vi "getImage.vi"(8 "error in (no error)":errorcluster, 10 "stop":bool, 11 "AndorIKonAcquisitor in":refnum<class "AndorIKonAcquisitor.lvclass">) -> (0 "error out":errorcluster, 2 "Array":path[](array[path]), 3 "AndorIKonAcquisitor out":refnum<class "AndorIKonAcquisitor.lvclass">)   [LabVIEW 2009, in "Hardware.lvlib" / "Channels.lvlib" / "AndorIKonAcquisitor.lvclass"]
uses:
  AndorIKonAcquisitor.lvclass
  <vilib>/vision/NI_Vision_Development_Module.lvlib
  Tools/Filing/FileSystem/FileSystem.lvclass
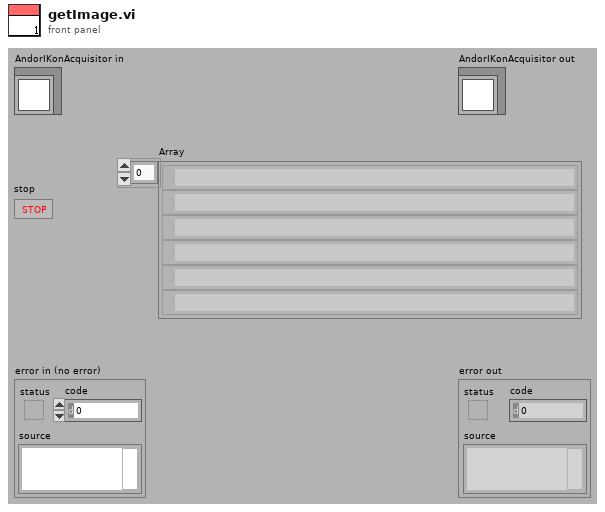
[diagram p1: front panel]
types:
  T1 = cluster{"Acquisition mode":dbl, "Readout Mode":dbl, "Gain":dbl}
  T2 = typedef "Error Code Enum typedef.ctl" = enum32{"N/A (0)", "DRV_ERROR_CODES", "DRV_SUCCESS", "DRV_VXDNOTINSTALLED", "DRV_ERROR_SCAN", "DRV_ERROR_CHECK_SUM", "DRV_ERROR_FILELOAD", "DRV_UNKNOWN_FUNC", "DRV_ERROR_VXD_INIT", "DRV_ERROR_ADDRESS", "DRV_ERROR_PAGELOCK", "DRV_ERROR_PAGEUNLOCK", "DRV_ERROR_BOARDTEST", "DRV_ERROR_ACK", "DRV_ERROR_UP_FIFO", "DRV_ERROR_PATTERN", "N/A (16)", "DRV_ACQUISITION_ERRORS", "DRV_ACQ_BUFFER", "DRV_ACQ_DOWNFIFO_FULL", "DRV_PROC_UNKONWN_INSTRUCTION", "DRV_ILLEGAL_OP_CODE", "DRV_KINETIC_TIME_NOT_MET", "DRV_ACCUM_TIME_NOT_MET", "DRV_NO_NEW_DATA", "N/A (25)", "DRV_SPOOLERROR", "N/A (27)", "N/A (28)", "N/A (29)", "N/A (30)", "N/A (31)", "N/A (32)", "DRV_TEMPERATURE_CODES", "DRV_TEMPERATURE_OFF", "DRV_TEMPERATURE_NOT_STABILIZED", "DRV_TEMPERATURE_STABILIZED", "DRV_TEMPERATURE_NOT_REACHED", "DRV_TEMPERATURE_OUT_RANGE", "DRV_TEMPERATURE_NOT_SUPPORTED", "DRV_TEMPERATURE_DRIFT", "N/A (41)", "N/A (42)", "N/A (43)", "N/A (44)", "N/A (45)", "N/A (46)", "N/A (47)", "N/A (48)", "DRV_GENERAL_ERRORS", "DRV_INVALID_AUX", "DRV_COF_NOTLOADED", "DRV_FPGAPROG", "DRV_FLEXERROR", "DRV_GPIBERROR", "N/A (55)", "N/A (56)", "N/A (57)", "N/A (58)", "N/A (59)", "N/A (60)", "N/A (61)", "N/A (62)", "N/A (63)", "DRV_DATATYPE", "DRV_DRIVER_ERRORS", "DRV_P1INVALID", "DRV_P2INVALID", "DRV_P3INVALID", "DRV_P4INVALID", "DRV_INIERROR", "DRV_COFERROR", "DRV_ACQUIRING", "DRV_IDLE", "DRV_TEMPCYCLE", "DRV_NOT_INITIALIZED", "DRV_P5INVALID", "DRV_P6INVALID", "DRV_INVALID_MODE", "DRV_INVALID_FILTER", "DRV_I2CERRORS", "DRV_I2CDEVNOTFOUND", "DRV_I2CTIMEOUT", "DRV_P7INVALID", "N/A (84)", "N/A (85)", "N/A (86)", "N/A (87)", "N/A (88)", "N/A (89)", "DRV_IOCERROR", "DRV_VRMVERSIONERROR"}
  T3 = cluster{"Vertical Binning":dbl, "Horizontal Binning":dbl, "SubArea Height":dbl, "SubAreaWidth":dbl, "Offset":dbl, "Number of Tracks":dbl, "Track Positions":cluster{"Top":dbl, "Bottom ":dbl}[], "subArea Coordinate":dbl[]}
  T4 = typedef "IMAQ Image.ctl" = refnum<image>
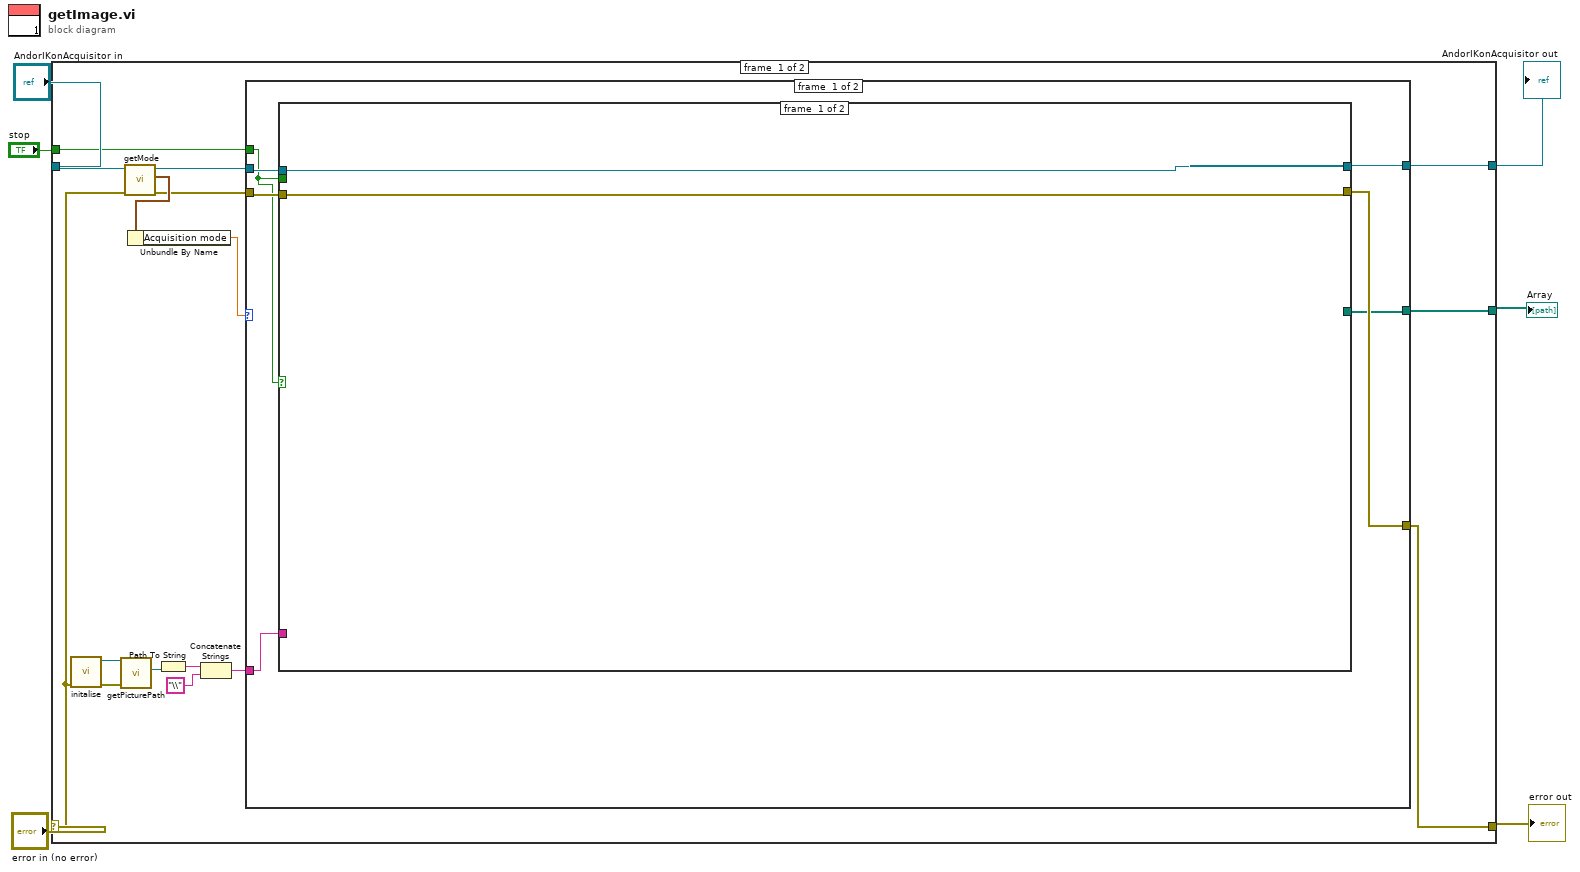
[diagram p0: block diagram]
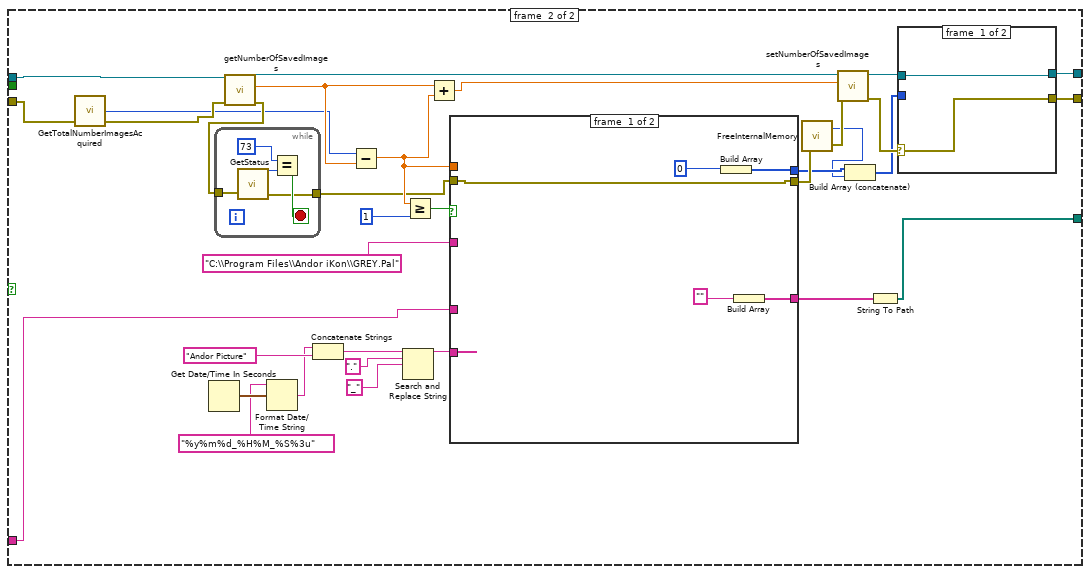
[diagram p2: hidden frame]
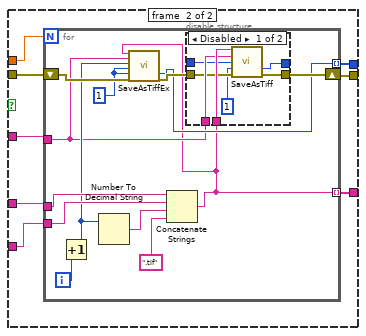
[diagram p3: hidden frame]
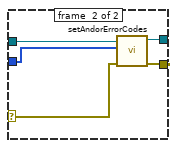
[diagram p5: hidden frame]
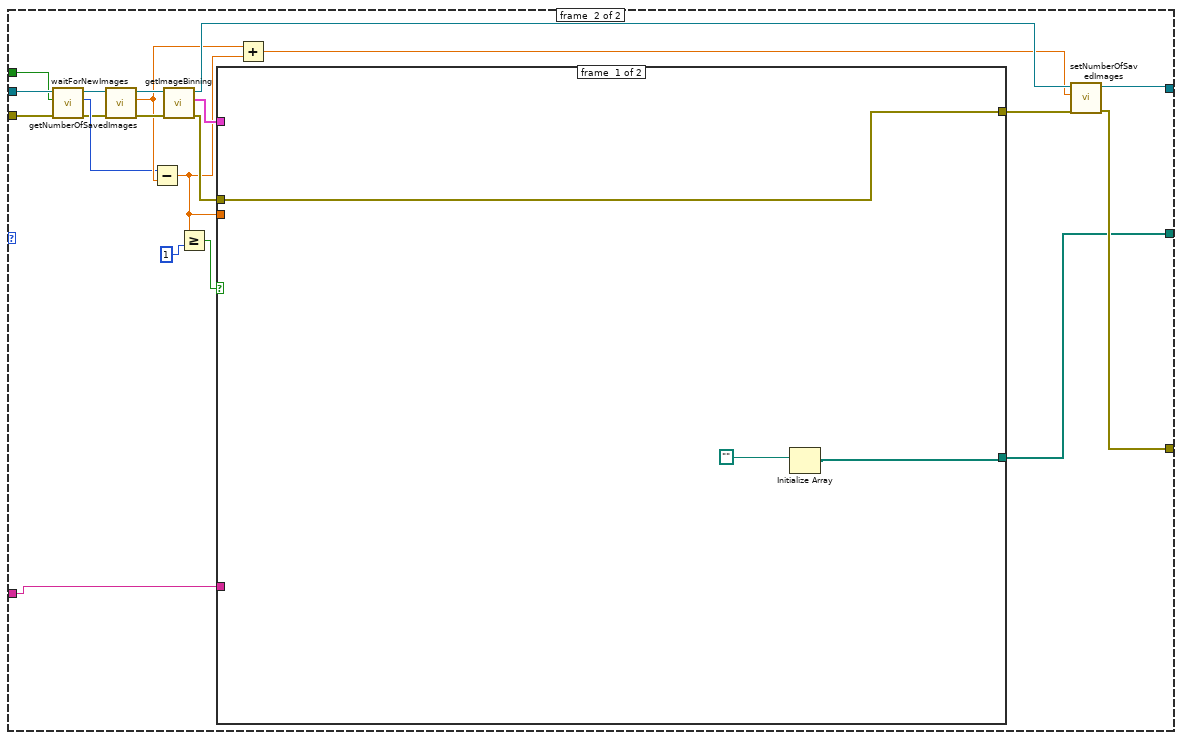
[diagram p6: hidden frame]
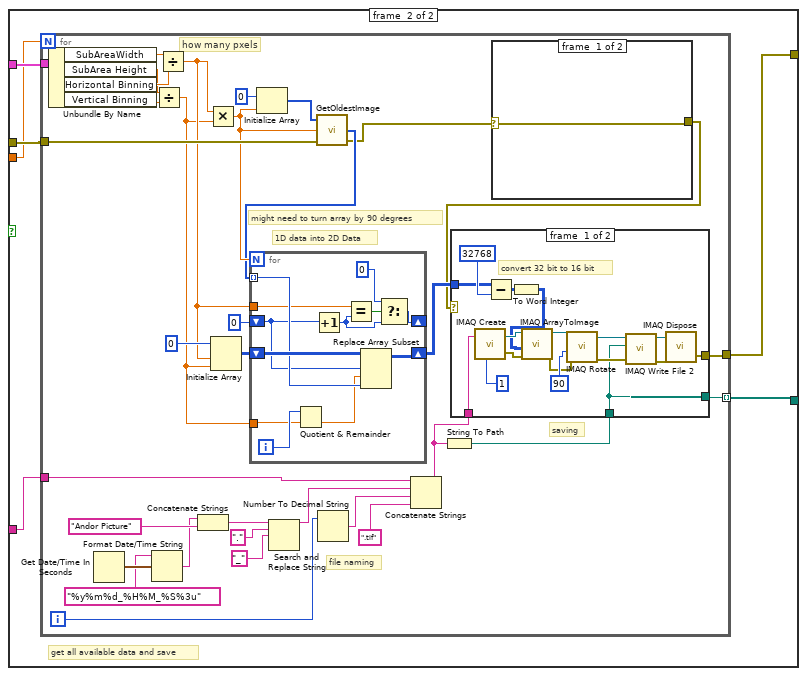
[diagram p7: hidden frame]
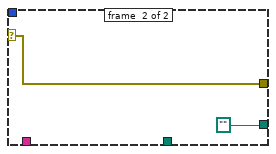
[diagram p8: hidden frame]
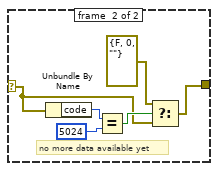
[diagram p9: hidden frame]
diagram:
  n1 = case shown="No Error" "error in (no error)" {
    selector: "error in (no error)" -> [w8 w213]
    tunnel: [w21 w213] -> w5
    tunnel: "AndorIKonAcquisitor in" -> [w19 w212]
    tunnel: [w22 w212] -> w3
    tunnel: [w20 _] -> w2
    tunnel: "stop" -> [w14 _]
    frame #0 {
      n2 = call "initalise.vi"("error in (no error)"=w8) -> ("error out"=w10:errorcluster, "FileSystem out"=w9:refnum<class "FileSystem.lvclass">)  [unwired: 9 in]
      n3 = call "getPicturePath.vi"("error in (no error)"=w10, "FileSystem in"=w9) -> ("PicturePath"=w11:path)  [unwired: 7 in, 2 out]
      n4 = call-dynamic "getMode.vi"("error in (no error)"=w8, "CameraAcquisitor.lvclass in"=w19) -> ("error out"=w17:errorcluster, "Mode"=w18:T1, "CameraAcquisitor.lvclass out"=w16:refnum<class "AndorIKonAcquisitor.lvclass">)  [unwired: 7 in]
      n5 = Unbundle By Name(w18) -> ("Acquisition mode"=w15:dbl)
      n6 = Path To String(path=w11) -> (string=w12:string)
      n7 = Concatenate Strings(w12, "\\") -> (w7:string)
      n8 = case shown="5" w15 {
        tunnel: [w29 w120] -> w22
        tunnel: [w28 w121] -> w21
        tunnel: [w27 w119] -> w20
        tunnel: w17 -> [w25 w112]
        tunnel: w16 -> [w26 w113]
        tunnel: w14 -> [w24 w111]
        tunnel: w7 -> [w23 w110]
        frame #0 {
          n9 = case shown="True" w24 {
            tunnel: [w31 w64] -> w29
            tunnel: [w30 w63] -> w28
            tunnel: [_ w58] -> w27
            tunnel: w26 -> [w31 w41]
            tunnel: w24 -> [_ _]
            tunnel: w25 -> [w30 w38]
            tunnel: w23 -> [_ w32]
            frame #0 {
            }
            frame #1 {
              n10 = call <userlib>:"GetTotalNumberImagesAcquired.vi"("error in (no error)"=w38) -> ("error out"=w40:errorcluster, "index"=w39:i32)  [unwired: 2 in, 1 out]
              n11 = Get Date/Time In Seconds() -> (seconds since 1Jan1904=w62:timestamp)
              n12 = call "getNumberOfSavedImages.vi"("error in (no error)"=w40, "AndorIKonAcquisitor.lvclass in"=w41) -> ("error out"=w44:errorcluster, "NumberOfSavedImages"=w42:dbl, "AndorIKonAcquisitor.lvclass out"=w48:refnum<class "AndorIKonAcquisitor.lvclass">)  [unwired: 7 in]
              n13 = while {
                tunnel: [w66] -> w43
                tunnel: w44 -> [w65]
                stop <- w67 stop-if-true
                n14 = call <userlib>:"GetStatus.vi"("error in (no error)"=w65) -> ("error out"=w66:errorcluster, "status"=w68:T2)  [unwired: 2 in, 1 out]
                n15 = Equal?(x=73, y=w68) -> (x = y?=w67:bool)
              }
              n16 = Format Date/Time String(time format string (%c)="%y%m%d_%H%M_%S%3u", seconds (now)=w62) -> (date/time string=w59:string)  [unwired: 1 in]
              n17 = Concatenate Strings(w59, "Andor Picture") -> (w57:string)
              n18 = Subtract(x=w39, y=w42) -> (x-y=w45:dbl)
              n19 = Search and Replace String(input string=w57, search string=".", replace string="_") -> (result string=w54:string)  [unwired: 5 in, 3 out]
              n20 = Greater Or Equal?(x=w45, y=1) -> (x >= y?=w50:bool)
              n21 = Add(x=w42, y=w45) -> (x+y=w47:dbl)
              n22 = case shown="True" w50 {
                tunnel: "C:\\Program Files\\Andor iKon\\GREY.Pal" -> [_ w82]
                tunnel: w32 -> [_ w81]
                tunnel: w54 -> [_ w80]
                tunnel: [w70 w79] -> w53
                tunnel: w43 -> [w72 w76]
                tunnel: w45 -> [_ w78]
                tunnel: [w73 w77] -> w35
                tunnel: [w72 w75] -> w37
                frame #0 {
                  n23 = Build Array(0) -> (w73:i32[])
                  n24 = Build Array("") -> (w70:string[])
                }
                frame #1 {
                  n25 = for {
                    N: w78 -> [_]
                    tunnel: w82 -> [w84]
                    tunnel: w81 -> [w95]
                    tunnel: w80 -> [w93]
                    tunnel: [w83] -> w79 mode=indexing
                    tunnel: [w85] -> w77 mode=indexing
                    shift-right: [w91] -> w75
                    shift-left: w76 -> [w89]
                    i -> [w90]
                    w86 = 1
                    n26 = Increment(x=w90) -> (x+1=w87:i32)
                    n27 = Number To Decimal String(number=w87) -> (decimal integer string=w94:string)  [unwired: 1 in]
                    n28 = Concatenate Strings(w95, w93, w94, ".tif") -> (w83:string)
                    n29 = call <userlib>:"SaveAsTiffEx.vi"("path"=w83, "palette"=w84, "position"=w87, "type"=w86, "mode"=w86, "error in (no error)"=w89) -> ("DLL error code"=w85:u32, "error out"=w88:errorcluster)  [unwired: 12 in]
                    n30 = disable-structure shown="Disabled" {
                      disable-tunnel: [w102 _] -> _
                      disable-tunnel: w83 -> [w101 _]
                      disable-tunnel: w84 -> [w100 _]
                      disable-tunnel: [w99 _] -> w91
                      disable-tunnel: w88 -> [w98 _]
                      disable-tunnel: _ -> [w96 _]
                      frame #0 {
                        n31 = call <userlib>:"SaveAsTiff.vi"("path"=w101, "palette"=w100, "position"=w96, "type"=1, "error in (no error)"=w98) -> ("DLL error code"=w102:u32, "error out"=w99:errorcluster)  [unwired: 9 in]
                      }
                      frame #1 {
                      }
                    }
                  }
                }
              }
              n32 = call <userlib>:"FreeInternalMemory.vi"("error in (no error)"=w37) -> ("error out"=w36:errorcluster, "DLL error code"=w34:u32)  [unwired: 1 in]
              n33 = call "setNumberOfSavedImages.vi"("error in (no error)"=w36, "NumberOfSavedImages"=w47, "AndorIKonAcquisitor.lvclass in"=w48) -> ("error out"=w46:errorcluster, "AndorIKonAcquisitor.lvclass out"=w49:refnum<class "AndorIKonAcquisitor.lvclass">)  [unwired: 7 in]
              n34 = Build Array (concatenate)(w35, w34) -> (w33:u32[])
              n35 = String To Path(string=w53) -> (path=w58:path[])
              n36 = case shown="Error" w46 {
                selector: w46 -> [w104 w109]
                tunnel: w49 -> [w103 w106]
                tunnel: [w103 w107] -> w64
                tunnel: [w104 w108] -> w63
                tunnel: w33 -> [_ w105]
                frame #0 {
                }
                frame #1 {
                  n37 = call-dynamic "setAndorErrorCodes.vi"("error in (no error)"=w109, "Andor Error Codes"=w105, "AndorIKonAcquisitor.lvclass in"=w106) -> ("error out"=w108:errorcluster, "AndorIKonAcquisitor.lvclass out"=w107:refnum<class "AndorIKonAcquisitor.lvclass">)  [unwired: 7 in]
                }
              }
            }
          }
        }
        frame #1 {
          n38 = call-dynamic "waitForNewImages.vi"("error in (no error)"=w112, "stop"=w111, "AndorIKonAcquisitor in"=w113) -> ("error out"=w116:errorcluster, "IndexOfNewImages"=w117:i32, "AndorIKonAcquisitor out"=w118:refnum<class "AndorIKonAcquisitor.lvclass">)  [unwired: 6 in]
          n39 = call "getNumberOfSavedImages.vi"("error in (no error)"=w116, "AndorIKonAcquisitor.lvclass in"=w118) -> ("error out"=w126:errorcluster, "NumberOfSavedImages"=w124:dbl, "AndorIKonAcquisitor.lvclass out"=w127:refnum<class "AndorIKonAcquisitor.lvclass">)  [unwired: 7 in]
          n40 = Subtract(x=w117, y=w124) -> (x-y=w114:dbl)
          n41 = call-dynamic "getImageBinning.vi"("error in (no error)"=w126, "CameraAcquisitor.lvclass in"=w127) -> ("error out"=w129:errorcluster, "Image Binning"=w128:T3, "CameraAcquisitor.lvclass out"=w125:refnum<class "AndorIKonAcquisitor.lvclass">)  [unwired: 7 in]
          n42 = Greater Or Equal?(x=w114, y=1) -> (x >= y?=w130:bool)
          n43 = case shown="True" w130 {
            tunnel: w129 -> [w133 w139]
            tunnel: w128 -> [_ w138]
            tunnel: w114 -> [_ w135]
            tunnel: [w133 w137] -> w122
            tunnel: [w131 w136] -> w119
            tunnel: w110 -> [_ w134]
            frame #0 {
              n44 = Initialize Array(path "") -> (w131:path[])  [unwired: 1 in]
            }
            frame #1 {
              # "get all available data and save"
              n45 = for {
                N: w135 -> [_]
                tunnel: w139 -> [w173]
                tunnel: w138 -> [w172]
                tunnel: [w159] -> w137
                tunnel: [w147] -> w136 mode=indexing
                tunnel: w134 -> [w140]
                i -> [w156]
                # "might need to turn array by 90 degrees"
                # "saving"
                # "file naming"
                # "how many pxels"
                # "1D data into 2D Data"
                n46 = Unbundle By Name(w172) -> ("SubAreaWidth"=w146:dbl, "SubArea Height"=w143:dbl, "Horizontal Binning"=w145:dbl, "Vertical Binning"=w142:dbl)
                n47 = Get Date/Time In Seconds() -> (seconds since 1Jan1904=w168:timestamp)
                n48 = Format Date/Time String(time format string (%c)="%y%m%d_%H%M_%S%3u", seconds (now)=w168) -> (date/time string=w165:string)  [unwired: 1 in]
                n49 = Divide(x=w143, y=w142) -> (x/y=w141:dbl)
                n50 = Divide(x=w146, y=w145) -> (x/y=w144:dbl)
                n51 = Concatenate Strings(w165, "Andor Picture") -> (w164:string)
                n52 = Multiply(x=w144, y=w141) -> (x*y=w155:dbl)
                n53 = Initialize Array(i16 0, w144, w141) -> (w169:i16[][])
                n54 = Initialize Array(u16 0, w155) -> (w158:u16[])
                n55 = Search and Replace String(input string=w164, search string=".", replace string="_") -> (result string=w154:string)  [unwired: 5 in, 3 out]
                n56 = call <userlib>:"GetOldestImage.vi"("error in (no error)"=w173, "size"=w155, "array"=w158) -> ("error out"=w149:errorcluster, "array"=w150:i32[])  [unwired: 1 out]
                n57 = for {
                  N: w155 -> [_]
                  tunnel: w150 -> [w203] mode=indexing
                  shift-right: [w204] -> _
                  shift-left: 0 -> [w201]
                  shift-right: [w211] -> w151
                  shift-left: w169 -> [w210]
                  tunnel: w141 -> [w208]
                  tunnel: w144 -> [w200]
                  i -> [w209]
                  n58 = Quotient & Remainder(x=w209, y=w208) -> (floor(x/y)=w202:dbl)  [unwired: 1 out]
                  n59 = Increment(x=w201) -> (x+1=w206:i32)
                  n60 = Equal?(x=w200, y=w206) -> (x = y?=w207:bool)
                  n61 = Replace Array Subset(array=w210, new element=w203, index (row)=w201, index (col)=w202) -> (w211:i16[][])
                  n62 = Select(t=0, s=w207, f=w206) -> (s? t:f=w204:i32)
                }
                n63 = Number To Decimal String(number=w156) -> (decimal integer string=w153:string)  [unwired: 1 in]
                n64 = Concatenate Strings(w140, w154, w153, ".tif") -> (w160:string)
                n65 = String To Path(string=w160) -> (path=w152:path)
                n66 = case shown="Error" w149 {
                  selector: w149 -> [w193 w196]
                  tunnel: [w193 w195] -> w148
                  frame #0 {
                  }
                  frame #1 {
                    # "no more data available yet"
                    n67 = Unbundle By Name(w196) -> ("code"=w199:i32)
                    n68 = Equal?(x=w199, y=5024) -> (x = y?=w197:bool)
                    n69 = Select(t=errorcluster {"status"=FALSE, "code"=0, "source"=""}, s=w197, f=w196) -> (s? t:f=w195:errorcluster)
                  }
                }
                n70 = case shown="No Error" w148 {
                  selector: w148 -> [_ w192]
                  tunnel: w160 -> [w189 _]
                  tunnel: [w188 w192] -> w159
                  tunnel: w152 -> [w180 _]
                  tunnel: w151 -> [w183 _]
                  tunnel: [w180 path ""] -> w147
                  frame #0 {
                    # "convert 32 bit to 16 bit"
                    n71 = call "IMAQ Create"("Image Name"=w189, "Image Type"=1) -> ("New Image"=w177:T4, "error out"=w176:errorcluster)  [unwired: 3 in]
                    n72 = Subtract(x=w183, y=32768) -> (x-y=w186:i32[][])
                    n73 = To Word Integer(number=w186) -> (16bit integer=w175:i16[][])
                    n74 = call "IMAQ ArrayToImage"("error in (no error)"=w176, "Image Pixels (I16)"=w175, "Image"=w177) -> ("error out"=w174:errorcluster, "Image Out"=w178:T4)  [unwired: 7 in]
                    n75 = call "IMAQ Rotate"("error in (no error)"=w174, "Angle (degrees)"=90, "Image Src"=w178) -> ("error out"=w182:errorcluster, "Image Dst Out"=w181:T4)  [unwired: 7 in]
                    n76 = call-poly "IMAQ Write File 2"("error in (no error)"=w182, "File Path"=w180, "Image"=w181) -> ("error out"=w185:errorcluster, "Image Out (duplicate)"=w184:T4)  [unwired: 7 in]
                    n77 = call "IMAQ Dispose"("Image"=w184, "error in (no error)"=w185) -> ("error out"=w188:errorcluster)  [unwired: 4 in]
                  }
                  frame #1 {
                  }
                }
              }
            }
          }
          n78 = Add(x=w124, y=w114) -> (x+y=w123:dbl)
          n79 = call "setNumberOfSavedImages.vi"("error in (no error)"=w122, "NumberOfSavedImages"=w123, "AndorIKonAcquisitor.lvclass in"=w125) -> ("error out"=w121:errorcluster, "AndorIKonAcquisitor.lvclass out"=w120:refnum<class "AndorIKonAcquisitor.lvclass">)  [unwired: 7 in]
        }
      }
    }
    frame #1 {
    }
  }
  "error out" <- w5
  "AndorIKonAcquisitor out" <- w3
  "Array" <- w2
